vi "123-1.vi"() -> ()   [LabVIEW 2015]
panel:
  out "Waveform Graph":dbl[][](graph)
  out "Waveform Chart":dbl[][](graph)
  out "Array 2":i32[](array[numeric])
  out "Array":i32[](array[numeric])
  in  "Numeric":i32=1
  out "element":dbl
  out "appended array":dbl[][](array[numeric])
  out "size(s)":i32
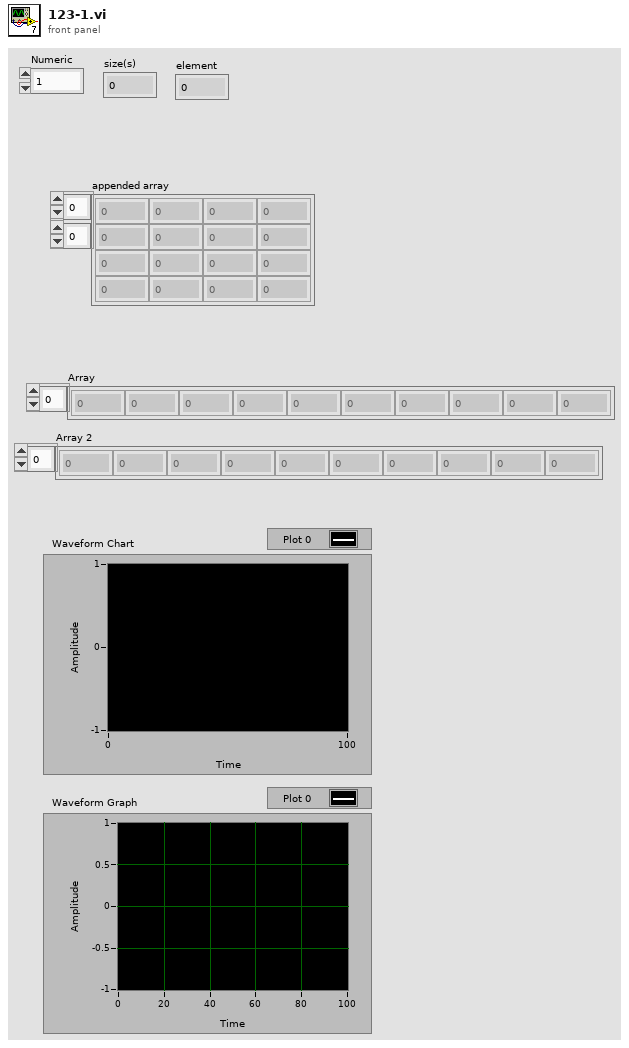
[diagram p1: front panel]
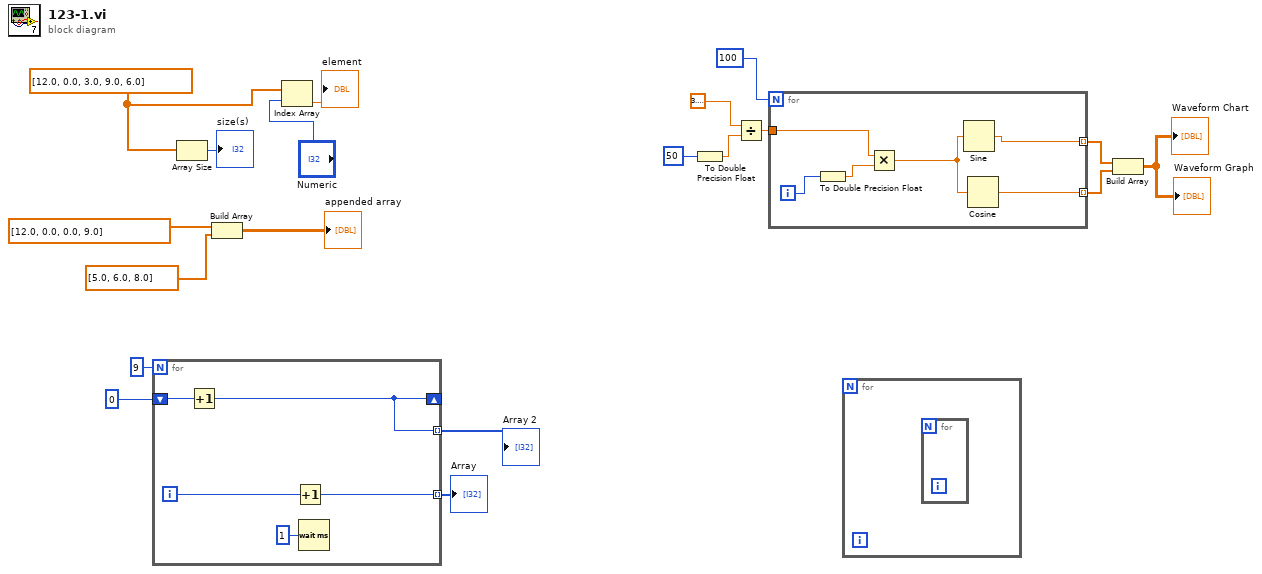
[diagram p0: block diagram]
diagram:
  w15 = dbl[] [12.0, 0.0, 3.0, 9.0, 6.0]
  n1 = for {
    N: 9 -> [_]
    shift-right: [w20] -> _
    shift-left: 0 -> [w24]
    tunnel: [w21] -> w10 mode=indexing
    tunnel: [w20] -> w9 mode=indexing
    i -> [w22]
    n2 = Increment(x=w24) -> (x+1=w20:i32)
    n3 = Increment(x=w22) -> (x+1=w21:i32)
    n4 = Wait (ms)(milliseconds to wait=u32 1) -> ()  [unwired: 1 out]
  }
  "Array" <- w10
  "Array 2" <- w9
  n5 = Array Size(array=w15) -> (size(s)=→"size(s)":i32)
  n6 = Build Array(dbl[] [12.0, 0.0, 0.0, 9.0], dbl[] [5.0, 6.0, 8.0]) -> (→"appended array":dbl[][])
  n7 = Index Array(array=w15, index="Numeric") -> (element=→"element":dbl)
  n8 = To Double Precision Float(number=50) -> (double precision float=w6:dbl)
  n9 = Divide(x=3.141592653589793, y=w6) -> (x/y=w4:dbl)
  n10 = for {
    N: 100 ("Numeric 2") -> [_]
    tunnel: w4 -> [w28]
    tunnel: [w26] -> w2 mode=indexing
    tunnel: [w25] -> w1 mode=indexing
    i -> [w29]
    n11 = To Double Precision Float(number=w29) -> (double precision float=w30:dbl)
    n12 = Multiply(x=w28, y=w30) -> (x*y=w27:dbl)
    n13 = Sine(x=w27) -> (sin(x)=w26:dbl)
    n14 = Cosine(x=w27) -> (cos(x)=w25:dbl)
  }
  n15 = for {
    n16 = for {
    }
  }
  n17 = Build Array(w2, w1) -> (→"Waveform Chart" →"Waveform Graph":dbl[][])
